vi "Emballage_BDD_lectures_tables.vi"(0 "Champ_resultat":string, 1 "num_piece":string, 3 "Champs-condition":string[](array[string]), 5 "Table_BDD":string, 7 "ID_ARTICLE?":bool, 9 "VALVE":string[](array[string]), 11 "entrée d'erreur (pas d'erreur)":errorcluster, 12 "ID_ARTICLE":string, 13 "Champ_ordre":string, 14 "valeur_condition":string[](array[string])) -> (4 "données":string[][](array[string]), 6 "info":string, 15 "sortie d'erreur":errorcluster)   [LabVIEW 2020]
uses:
  Modules/FS/60_FS_Controles/60_FS_SetGet.ctl
  <vilib>/addons/database/Connection.llb/DB Tools Open Connec (Path).vi
  <vilib>/addons/database/Connection.llb/Conn Execute.vi
  <vilib>/addons/database/Recordset.llb/Rec Fetch Recordset Data (R).vi
  <vilib>/addons/database/Recordset.llb/Rec Destroy - Connection.vi
  <vilib>/addons/database/NI_Database_API.lvlib
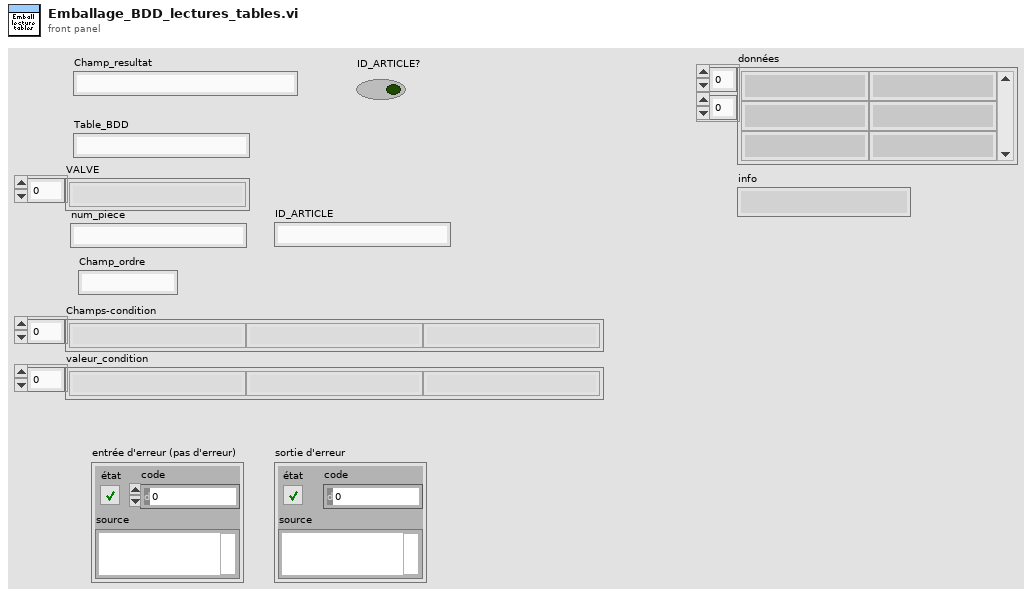
[diagram p1: front panel]
types:
  T1 = typedef "60_FS_SetGet.ctl" = enum16{"set", "get"}
  T2 = typedef "60_FS_CLT_Chemins.ctl" = cluster{"Racine_local":path, "Racine_reseau":path, "Racine_Support_Application":path, "Fichier_Journalisation":path, "Connexion_BDD_VSX":path, "Connexion_BDD_PLZ":path}
  T3 = typedef "NI_Database_API.lvlib/Conn ObjectReference.ctl" = refnum<k1>
  T4 = typedef "NI_Database_API.lvlib/Rec ObjectReference.ctl" = refnum<k1>
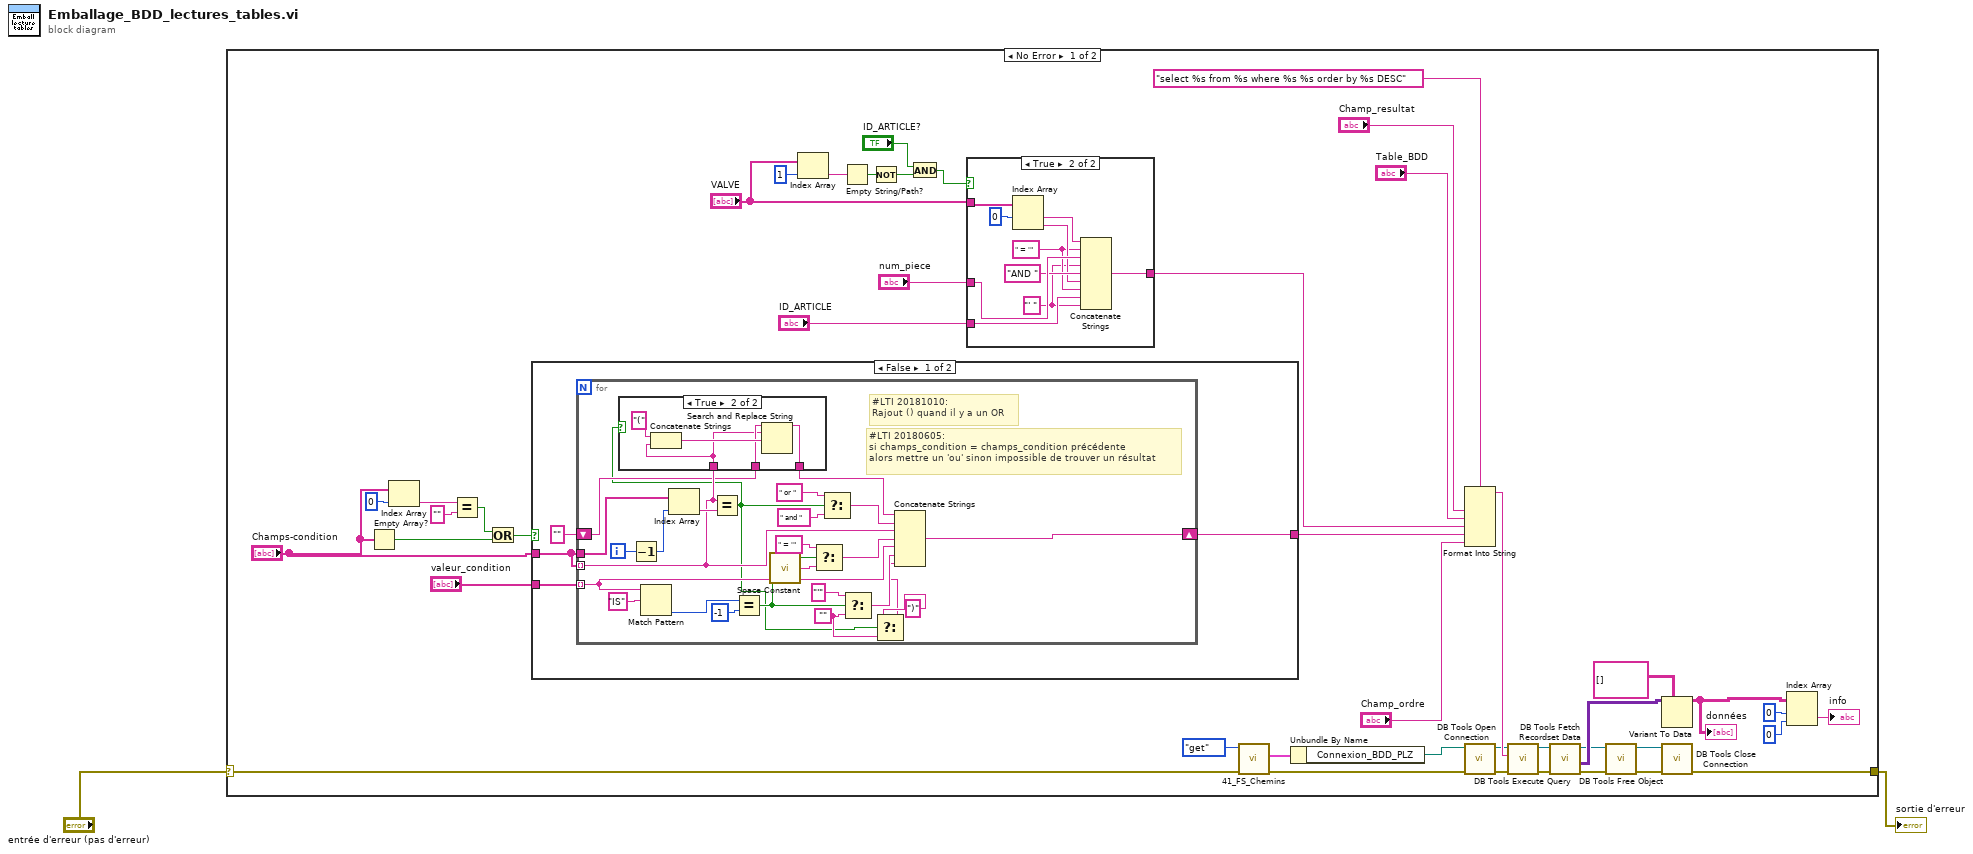
[diagram p0: block diagram]
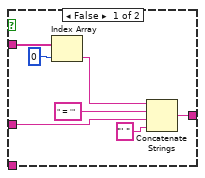
[diagram p2: hidden frame]
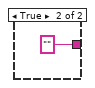
[diagram p4: hidden frame]
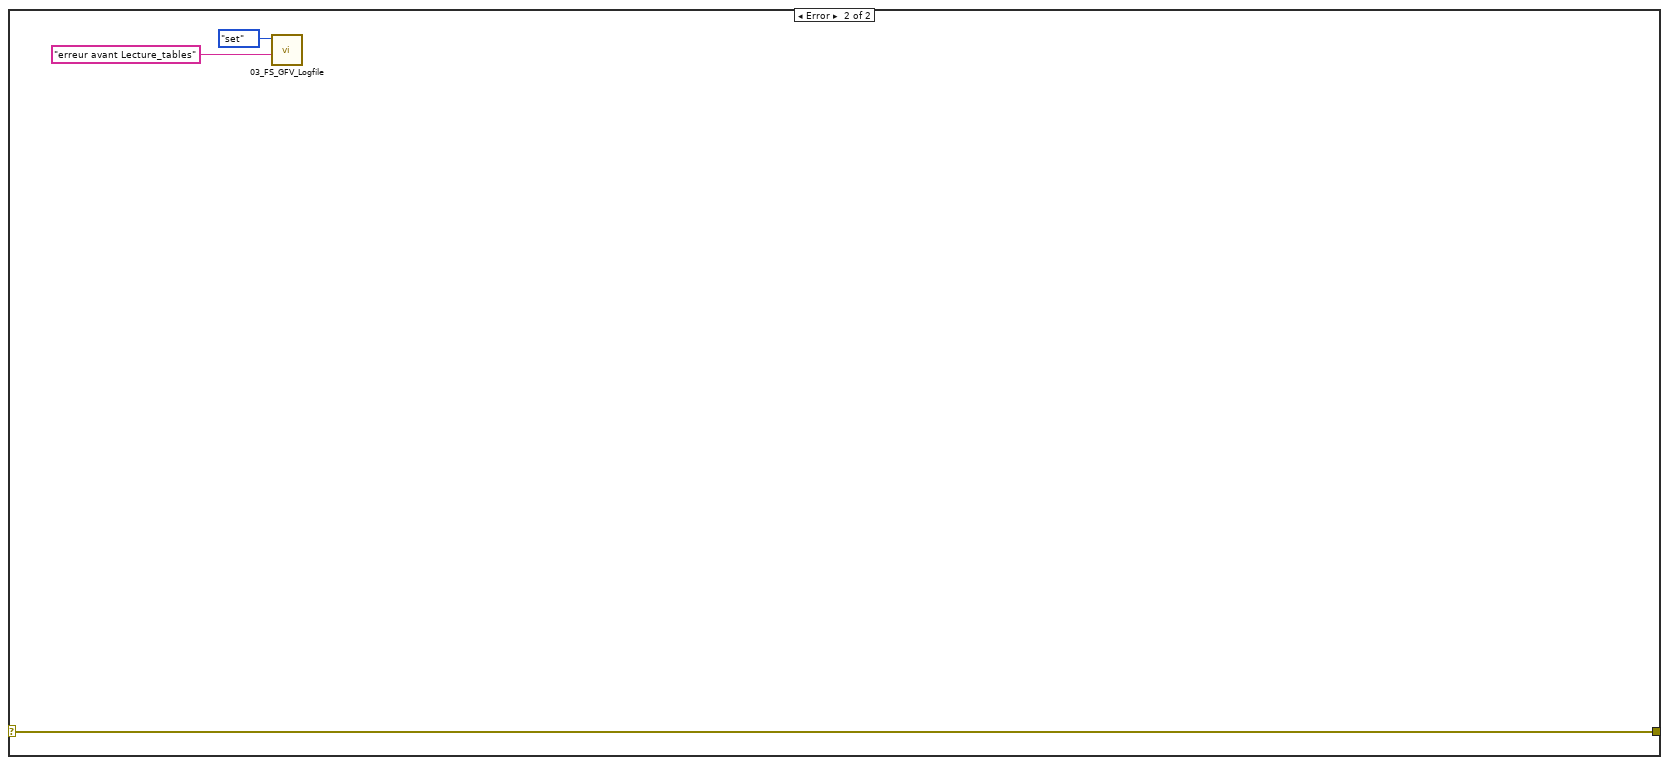
[diagram p5: hidden frame]
diagram:
  n1 = case shown="No Error" "entrée d'erreur (pas d'erreur)" {
    selector: "entrée d'erreur (pas d'erreur)" -> [w13 w102]
    tunnel: [w12 w102] -> w1
    frame No Error {
      n2 = Empty Array?(array="Champs-condition") -> (empty?=w22:bool)
      n3 = Index Array(array="Champs-condition", index=0 ("indice")) -> (element=w18:string)
      n4 = Equal?(x=w18, y="") -> (x = y?=w15:bool)
      n5 = Or(x=w15, y=w22) -> (x .or. y?=w16:bool)
      n6 = case shown="False" w16 {
        tunnel: "Champs-condition" -> [w64 _]
        tunnel: "valeur_condition" -> [w65 _]
        tunnel: [w67 ""] -> w21
        frame False {
          n7 = for {
            shift-right: [w92] -> w67
            shift-left: "" -> [w70]
            tunnel: w65 -> [w84] mode=indexing
            tunnel: w64 -> [w71] mode=indexing
            tunnel: w64 -> [w91]
            i -> [w90]
            w73 = ""
            # "#LTI 20181010:\nRajout () quand il y a un OR"
            # "#LTI 20180605:\nsi champs_condition = champs_condition précédente\nalors mettre un 'ou' sinon impossible de trouver un résultat"
            n8 = Decrement(x=w90) -> (x-1=w89:i32)
            n9 = Match Pattern(string=w84, regular expression="IS" ("expression régulière")) -> (offset past match=w82:i32)  [unwired: 1 in, 3 out]
            n10 = Index Array(array=w91, index=w89) -> (element=w88:string)
            n11 = Equal?(x=w71, y=w88) -> (x = y?=w68:bool)
            n12 = case shown="True" w68 {
              tunnel: w71 -> [_ w94]
              tunnel: w70 -> [w93 w96]
              tunnel: [w93 w95] -> w69
              frame False {
              }
              frame True {
                n13 = Concatenate Strings("(" ("chaîne"), w94) -> (w98:string)
                n14 = Search and Replace String(input string=w96, search string=w94, replace string=w98) -> (result string=w95:string)  [unwired: 5 in, 3 out]
              }
            }
            n15 = Equal?(x=w82, y=-1) -> (x = y?=w77:bool)
            n16 = call <vilib>:"Space Constant.vi"() -> ("String"=w76:string)
            n17 = Select(t=" = '" ("chaîne"), s=w77, f=w76) -> (s? t:f=w80:string)
            n18 = Select(t=" or " ("chaîne"), s=w68, f=" and " ("chaîne")) -> (s? t:f=w87:string)
            n19 = Select(t="'" ("chaîne"), s=w77, f=w73) -> (s? t:f=w75:string)
            n20 = Select(t=")" ("chaîne"), s=w68, f=w73) -> (s? t:f=w72:string)
            n21 = Concatenate Strings(w69, w87, w71, w80, w84, w75, w72) -> (w92:string)
          }
        }
        frame True {
        }
      }
      n22 = Index Array(array="VALVE", index=1 ("indice")) -> (element=w3:string)
      n23 = Empty String/Path?(string/path=w3) -> (empty?=w7:bool)
      n24 = Not(x=w7) -> (.not. x?=w4:bool)
      n25 = And(x="ID_ARTICLE?", y=w4) -> (x .and. y?=w9:bool)
      n26 = case shown="True" w9 {
        tunnel: [w53 w54] -> w14
        tunnel: "VALVE" -> [w50 w61]
        tunnel: "num_piece" -> [w49 w60]
        tunnel: "ID_ARTICLE" -> [_ w56]
        frame False {
          n27 = Index Array(array=w50, index=0 ("indice")) -> (element=w48:string)
          n28 = Concatenate Strings(w48, " = '" ("chaîne"), w49, "' " ("chaîne")) -> (w53:string)
        }
        frame True {
          w55 = "' " ("chaîne")
          w57 = " = '" ("chaîne")
          n29 = Index Array(array=w61, index #1=0 ("indice")) -> (element #1=w63:string, element #2=w58:string)  [unwired: 1 in]
          n30 = Concatenate Strings(w63, w57, w60, w55, "AND " ("chaîne"), w58, w57, w56, w55) -> (w54:string)
        }
      }
      n31 = call "41_FS_Chemins.vi"("error in (no error)"=w13, "SetGet"=60_FS_SetGet."get") -> ("error out"=w45:errorcluster, "CLT_Chemins_out"=w41:T2)  [unwired: 8 in]
      n32 = Unbundle By Name(w41) -> ("Connexion_BDD_PLZ"=w43:path)
      n33 = Format Into String(format string="select %s from %s where %s %s order by %s DESC" ("chaîne de format"), "Champ_resultat", "Table_BDD", w14, w21, "Champ_ordre") -> (resulting string=w36:string)  [unwired: 2 in, 1 out]
      n34 = call-poly <vilib>:"DB Tools Open Connection.vi"("error in (no error)"=w45, "connection information"=w43) -> ("error out"=w26:errorcluster, "connection reference"=w25:T3)  [unwired: 6 in]
      n35 = call-poly <vilib>:"DB Tools Execute Query.vi"("error in (no error)"=w26, "SQL query"=w36, "connection reference"=w25) -> ("error out"=w29:errorcluster, "recordset reference"=w31:T4)  [unwired: 5 in]
      n36 = call-poly <vilib>:"DB Tools Fetch Recordset Data.vi"("error in (no error)"=w29, "recordset reference"=w31) -> ("error out"=w30:errorcluster, "recordset data"=w33:variant[][], "recordset reference out"=w32:T4)  [unwired: 3 in]
      n37 = call-poly <vilib>:"DB Tools Free Object.vi"("error in (no error)"=w30, "recordset reference"=w32) -> ("error out"=w27:errorcluster, "connection reference"=w28:T3)  [unwired: 8 in]
      n38 = Variant To Data(type=string[][] [], Variant=w33) -> (data=w37:string[][])  [unwired: 1 in, 1 out]
      "données" <- w37
      n39 = call <vilib>:"DB Tools Close Connection.vi"("error in (no error)"=w27, "connection reference"=w28) -> ("error out"=w12:errorcluster)  [unwired: 5 in]
      n40 = Index Array(array=w37, index (row)=0 ("indice (ligne)"), index (col)=0 ("indice désactivé (col)")) -> (element=→"info":string)
    }
    frame Error {
      n41 = call "03_FS_GFV_Logfile.vi"("Chaîne"="erreur avant Lecture_tables", "States"=60_FS_SetGet."set") -> ()  [unwired: 8 in, 2 out]
    }
  }
  "sortie d'erreur" <- w1
